vi "rsscope_core_global.vi"() -> ()   [LabVIEW 2018] (continued)
"Data Type"=0, "Command"="SENS:SOUR", "Access"=2, "Range Table"="rsscope_rngIntExt", "Read Callback"="", "Write Callback"="", "Supported Models"="", "Instrument Options"="B4", "Flags"=0, "Help"="Enables the use of the external reference signal instead of the internal OCXO reference.\n\nAvailable Repeated Capabilities:\nNone\n\nRemote-control command(s):\nSENSe[:ROSCillator]:SOURce"}, {"Level"=2, "Class Only"=FALSE, "Identifier"="RSSCOPE_ATTR_REF_OSCILLATOR_FREQUENCY", "Descriptive Name"="Ref Oscillator Frequency", "Data Type"=1, "Command"="SENS:EXT:FREQ", "Access"=2, "Range Table"="rsscope_rngExtOscFreq", "Read Callback"="", "Write Callback"="", "Supported Models"="", "Instrument Options"="B4", "Flags"=0, "Help"="Sets the frequency of an external reference input signal that is connected to the external reference input on the rear panel.\n\nNote: Increment is 1e+6 Hz.\n\nAvailable Repeated Capabilities:\nNone\n\nRemote-control command(s):\nSENSe[:ROSCillator]:EXTernal:FREQuency"}, {"Level"=1, "Class Only"=TRUE, "Identifier"="", "Descriptive Name"="Probe", "Data Type"=0, "Command"="", "Access"=0, "Range Table"="", "Read Callback"="", "Write Callback"="", "Supported Models"="", "Instrument Options"="", "Flags"=0, "Help"="This class contains attributes that configure the probe subsystem."}, {"Level"=2, "Class Only"=FALSE, "Identifier"="RSSCOPE_ATTR_PROBE_STATE", "Descriptive Name"="Probe State", "Data Type"=0, "Command"="PROB{Channel}:SET:STAT?", "Access"=0, "Range Table"="rsscope_rngProbeState", "Read Callback"="", "Write Callback"="", "Supported Models"="", "Instrument Options"="", "Flags"=0, "Help"="Queries if the probe at the specified input channel is active (detected) or not active (not detected). To switch the probe on, use attribute RSSCOPE_ATTR_CHANNEL_ENABLED.\n\nAvailable Repeated Capabilities:\nChannel: CH1, CH2, CH3, CH4, CHExt\r\n\nRemote-control command(s):\nPROBe<m>:SETup:STATe?"}, {"Level"=2, "Class Only"=FALSE, "Identifier"="RSSCOPE_ATTR_PROBE_TYPE", "Descriptive Name"="Probe Type", "Data Type"=2, "Command"="PROB{Channel}:SET:TYPE?", "Access"=0, "Range Table"="", "Read Callback"="", "Write Callback"="", "Supported Models"="", "Instrument Options"="", "Flags"=0, "Help"="Queries the type of the probe.\n\nAvailable Repeated Capabilities:\nChannel: CH1, CH2, CH3, CH4, CHExt\r\n\nRemote-control command(s):\nPROBe<m>:SETup:TYPE?"}, {"Level"=2, "Class Only"=FALSE, "Identifier"="RSSCOPE_ATTR_PROBE_NAME", "Descriptive Name"="Probe Name", "Data Type"=2, "Command"="PROB{Channel}:SET:NAME?", "Access"=0, "Range Table"="", "Read Callback"="", "Write Callback"="", "Supported Models"="", "Instrument Options"="", "Flags"=0, "Help"="Queries the name of the probe.\n\nAvailable Repeated Capabilities:\nChannel: CH1, CH2, CH3, CH4, CHExt\r\n\nRemote-control command(s):\nPROBe<m>:SETup:NAME?"}, {"Level"=2, "Class Only"=FALSE, "Identifier"="RSSCOPE_ATTR_PROBE_INPUT_IMPEDANCE", "Descriptive Name"="Probe Input Impedance", "Data Type"=1, "Command"="PROB{Channel}:SET:IMP?", "Access"=0, "Range Table"="", "Read Callback"="", "Write Callback"="", "Supported Models"="", "Instrument Options"="", "Flags"=0, "Help"="Queries the termination of the probe.\n\nAvailable Repeated Capabilities:\nChannel: CH1, CH2, CH3, CH4, CHExt\r\n\nRemote-control command(s):\nPROBe<m>:SETup:IMPedance?"}, {"Level"=2, "Class Only"=FALSE, "Identifier"="RSSCOPE_ATTR_PROBE_INPUT_CAPACITANCE", "Descriptive Name"="Probe Input Capacitance", "Data Type"=1, "Command"="PROB{Channel}:SET:CAP?", "Access"=0, "Range Table"="", "Read Callback"="", "Write Callback"="", "Supported Models"="", "Instrument Options"="", "Flags"=0, "Help"="Queries the input capacitance of the probe.\n\nAvailable Repeated Capabilities:\nChannel: CH1, CH2, CH3, CH4, CHExt\r\n\nRemote-control command(s):\nPROBe<m>:SETup:CAPacitance?"}, {"Level"=2, "Class Only"=FALSE, "Identifier"="RSSCOPE_ATTR_PROBE_ATTENUATION", "Descriptive Name"="Probe Attenuation", "Data Type"=1, "Command"="PROB{Channel}:SET:ATT?", "Access"=0, "Range Table"="", "Read Callback"="", "Write Callback"="", "Supported Models"="", "Instrument Options"="", "Flags"=0, "Help"="Queries the attenuation of the probe.\n\nAvailable Repeated Capabilities:\nChannel: CH1, CH2, CH3, CH4, CHExt\r\n\nRemote-control command(s):\nPROBe<m>:SETup:ATTenuation[:AUTO]?"}, {"Level"=2, "Class Only"=FALSE, "Identifier"="RSSCOPE_ATTR_PROBE_BANDWIDTH", "Descriptive Name"="Probe Bandwidth", "Data Type"=1, "Command"="PROB{Channel}:SET:BANDwidth?", "Access"=0, "Range Table"="", "Read Callback"="", "Write Callback"="", "Supported Models"="", "Instrument Options"="", "Flags"=0, "Help"="Queries the bandwidth of the probe.\n\nAvailable Repeated Capabilities:\nChannel: CH1, CH2, CH3, CH4, CHExt\r\n\nRemote-control command(s):\nPROBe<m>:SETup:BANDwidth?"}, {"Level"=2, "Class Only"=FALSE, "Identifier"="RSSCOPE_ATTR_PROBE_SET_OFFSET_TO_MEAN", "Descriptive Name"="Probe Set Offset To Mean", "Data Type"=4, "Command"="PROB{Channel}:SET:OFFS:TOM", "Access"=1, "Range Table"="", "Read Callback"="", "Write Callback"="", "Supported Models"="", "Instrument Options"="", "Flags"=1, "Help"="Performs an automatic compensation for a DC component of the specified input signal using the result of a background mean measurement.\n\nAvailable Repeated Capabilities:\nChannel: CH1, CH2, CH3, CH4, CHExt\r\n\nRemote-control command(s):\nPROBe<m>:SETup:OFFSet:TOMean"}, {"Level"=2, "Class Only"=FALSE, "Identifier"="RSSCOPE_ATTR_PROBE_DEGAUSS", "Descriptive Name"="Probe Degauss", "Data Type"=4, "Command"="PROB{Channel}:SET:DEG", "Access"=1, "Range Table"="", "Read Callback"="", "Write Callback"="", "Supported Models"="", "Instrument Options"="", "Flags"=0, "Help"="Demagnetizes the core if it has been magnetized by switching the power on and off, or by an excessive input. Always carry out demagnetizing before measurement. The demagnetizing process takes about one second.\n\nAvailable Repeated Capabilities:\nChannel: CH1, CH2, CH3, CH4, CHExt\r\n\nRemote-control command(s):\nPROBe<m>:SETup:DEGauss"}, {"Level"=2, "Class Only"=FALSE, "Identifier"="RSSCOPE_ATTR_PROBE_AUTO_ZERO", "Descriptive Name"="Probe Auto Zero", "Data Type"=4, "Command"="PROB{Channel}:SET:OFFS:AZER", "Access"=1, "Range Table"="", "Read Callback"="", "Write Callback"="", "Supported Models"="", "Instrument Options"="", "Flags"=1, "Help"="Performs an automatic correction of the zero error. If the DUT is ground-referenced, the Auto Zero function can improve the measurement results.\n\nAvailable Repeated Capabilities:\nChannel: CH1, CH2, CH3, CH4, CHExt\r\n\nRemote-control command(s):\nPROBe<m>:SETup:OFFSet:AZERo"}, {"Level"=2, "Class Only"=FALSE, "Identifier"="RSSCOPE_ATTR_PROBE_USE_AUTO_ZERO", "Descriptive Name"="Probe Use Auto Zero", "Data Type"=3, "Command"="PROB{Channel}:SET:OFFS:USE", "Access"=2, "Range Table"="", "Read Callback"="", "Write Callback"="", "Supported Models"="", "Instrument Options"="", "Flags"=0, "Help"="Includes the AutoZero offset in measurement results.\n\nAvailable Repeated Capabilities:\nChannel: CH1, CH2, CH3, CH4, CHExt\r\n\nRemote-control command(s):\nPROBe<m>:SETup:OFFSet:USEautozero"}, {"Level"=2, "Class Only"=FALSE, "Identifier"="RSSCOPE_ATTR_PROBE_ZERO_ADJUST_VALUE", "Descriptive Name"="Probe Zero Adjust Value", "Data Type"=1, "Command"="PROB{Channel}:SET:OFFS:ZADJ", "Access"=2, "Range Table"="RsScope_rngProbeZeroAdjustValue", "Read Callback"="", "Write Callback"="", "Supported Models"="", "Instrument Options"="", "Flags"=0, "Help"="Set the waveform to zero position. It corrects the effect of a voltage offset or temperature drift.\n\nAvailable Repeated Capabilities:\nChannel: CH1, CH2, CH3, CH4, CHExt\r\n\nRemote-control command(s):\nPROBe<m>:SETup:OFFSet:ZADJust"}, {"Level"=2, "Class Only"=FALSE, "Identifier"="RSSCOPE_ATTR_PROBE_SAVE_TO_PROBE", "Descriptive Name"="Probe Save To Probe", "Data Type"=4, "Command"="PROB{Channel}:SET:OFFS:STPR", "Access"=1, "Range Table"="", "Read Callback"="", "Write Callback"="", "Supported Models"="", "Instrument Options"="", "Flags"=0, "Help"="Saves the zero adjust value in the probe box. If you connect the probe to another channel or to another R&S RTx oscilloscope, the value is read out again.\n\nAvailable Repeated Capabilities:\nChannel: CH1, CH2, CH3, CH4, CHExt\r\n\nRemote-control command(s):\nPROBe<m>:SETup:OFFSet:STPRobe"}, {"Level"=2, "Class Only"=FALSE, "Identifier"="RSSCOPE_ATTR_PROBE_MICRO_BUTTON_ACTION", "Descriptive Name"="Probe Micro Button Action", "Data Type"=0, "Command"="PROB{Channel}:SET:MODE", "Access"=2, "Range Table"="rsscope_rngProbeButtonAction", "Read Callback"="", "Write Callback"="", "Supported Models"="", "Instrument Options"="", "Flags"=0, "Help"="Select the action that is started with the micro button on the probe head.\n\nAvailable Repeated Capabilities:\nChannel: CH1, CH2, CH3, CH4, CHExt\r\n\nRemote-control command(s):\nPROBe<m>:SETup:MODE"}, {"Level"=2, "Class Only"=FALSE, "Identifier"="RSSCOPE_ATTR_PROBE_SOFTWARE_VERSION", "Descriptive Name"="Probe Software Version", "Data Type"=2, "Command"="PROB{Channel}:ID:SWV?", "Access"=0, "Range Table"="", "Read Callback"="", "Write Callback"="", "Supported Models"="", "Instrument Options"="", "Flags"=0, "Help"="Queries the version of the probe firmware.\n\nAvailable Repeated Capabilities:\nChannel: CH1, CH2, CH3, CH4, CHExt\r\n\nRemote-control command(s):\nPROBe<m>:ID:SWVersion?"}, {"Level"=2, "Class Only"=FALSE, "Identifier"="RSSCOPE_ATTR_PROBE_PRODUCTION_DATE", "Descriptive Name"="Probe Production Date", "Data Type"=2, "Command"="PROB{Channel}:ID:PRD?", "Access"=0, "Range Table"="", "Read Callback"="", "Write Callback"="", "Supported Models"="", "Instrument Options"="", "Flags"=0, "Help"="Queries the production date of the probe.\n\nAvailable Repeated Capabilities:\nChannel: CH1, CH2, CH3, CH4, CHExt\r\n\nRemote-control command(s):\nPROBe<m>:ID:PRDate?"}, {"Level"=2, "Class Only"=FALSE, "Identifier"="RSSCOPE_ATTR_PROBE_PART_NUMBER", "Descriptive Name"="Probe Part Number", "Data Type"=2, "Command"="PROB{Channel}:ID:PART?", "Access"=0, "Range Table"="", "Read Callback"="", "Write Callback"="", "Supported Models"="", "Instrument Options"="", "Flags"=0, "Help"="Queries the R&S part number of the probe.\n\nAvailable Repeated Capabilities:\nChannel: CH1, CH2, CH3, CH4, CHExt\r\n\nRemote-control command(s):\nPROBe<m>:ID:PARTnumber?"}, {"Level"=2, "Class Only"=FALSE, "Identifier"="RSSCOPE_ATTR_PROBE_SERIAL_NUMBER", "Descriptive Name"="Probe Serial Number", "Data Type"=2, "Command"="PROB{Channel}:ID:SRN?", "Access"=0, "Range Table"="", "Read Callback"="", "Write Callback"="", "Supported Models"="", "Instrument Options"="", "Flags"=0, "Help"="Queries the serial number of the probe.\n\nAvailable Repeated Capabilities:\nChannel: CH1, CH2, CH3, CH4, CHExt\r\n\nRemote-control command(s):\nPROBe<m>:ID:SRNumber?"}, {"Level"=2, "Class Only"=FALSE, "Identifier"="RSSCOPE_ATTR_PROBE_FIRMWARE_PATH", "Descriptive Name"="Probe Firmware Path", "Data Type"=2, "Command"="PROB{Channel}:SERV:FW:PATH", "Access"=2, "Range Table"="", "Read Callback"="", "Write Callback"="", "Supported Models"="", "Instrument Options"="", "Flags"=0, "Help"="Configures the path and file name of the update package.\n\nAvailable Repeated Capabilities:\nChannel: CH1, CH2, CH3, CH4, CHExt\r\n\nRemote-control command(s):\nPROBe<m>:SERVice:FW:PATH"}, {"Level"=2, "Class Only"=FALSE, "Identifier"="RSSCOPE_ATTR_PROBE_FIRMWARE_UPDATE", "Descriptive Name"="Probe Firmware Update", "Data Type"=4, "Command"="PROB{Channel}:SERV:FW:FLAS", "Access"=1, "Range Table"="", "Read Callback"="", "Write Callback"="", "Supported Models"="", "Instrument Options"="", "Flags"=0, "Help"="Starts the update of the probe firmware.\n\nAvailable Repeated Capabilities:\nChannel: CH1, CH2, CH3, CH4, CHExt\r\n\nRemote-control command(s):\nPROBe<m>:SERVice:FW:FLASh"}, {"Level"=2, "Class Only"=FALSE, "Identifier"="RSSCOPE_ATTR_PROBE_FIRMWARE_UPDATE_STATUS", "Descriptive Name"="Probe Firmware Update Status", "Data Type"=0, "Command"="PROB{Channel}:SERV:STAT?", "Access"=0, "Range Table"="rsscope_rngProbeFirmwareUpdateStatus", "Read Callback"="", "Write Callback"="", "Supported Models"="", "Instrument Options"="", "Flags"=0, "Help"="Queries the update status of the probe firmware.\n\nAvailable Repeated Capabilities:\nChannel: CH1, CH2, CH3, CH4, CHExt\r\n\nRemote-control command(s):\nPROBe<m>:SERVice:STATe?"}, {"Level"=2, "Class Only"=FALSE, "Identifier"="RSSCOPE_ATTR_PROBE_SELFTEST", "Descriptive Name"="Probe Selftest", "Data Type"=4, "Command"="PROB{Channel}:SERV:STES:RUN", "Access"=1, "Range Table"="", "Read Callback"="", "Write Callback"="", "Supported Models"="", "Instrument Options"="", "Flags"=0, "Help"="Starts the selftest of the probe connected to the specified channel input.\n\nAvailable Repeated Capabilities:\nChannel: CH1, CH2, CH3, CH4, CHExt\r\n\nRemote-control command(s):\nPROBe<m>:SERVice:STESt:RUN"}, {"Level"=2, "Class Only"=FALSE, "Identifier"="RSSCOPE_ATTR_PROBE_SELFTEST_STATUS", "Descriptive Name"="Probe Selftest Status", "Data Type"=0, "Command"="PROB{Channel}:SERV:STES:STAT?", "Access"=0, "Range Table"="rsscope_rngProbeSelftestStatus", "Read Callback"="", "Write Callback"="", "Supported Models"="", "Instrument Options"="", "Flags"=0, "Help"="Queries the status of a probe selftest for the specified channel input. When the selftest has finished, the status is passed or failed, otherwise it is undefined.\n\nAvailable Repeated Capabilities:\nChannel: CH1, CH2, CH3, CH4, CHExt\r\n\nRemote-control command(s):\nPROBe<m>:SERVice:STESt:STATus?"}, {"Level"=2, "Class Only"=FALSE, "Identifier"="RSSCOPE_ATTR_PROBE_DETECTION_MODE", "Descriptive Name"="Probe Detection Mode", "Data Type"=0, "Command"="PROB{Channel}:SET:ATT:MODE", "Access"=2, "Range Table"="rsscope_rngAutoManual", "Read Callback"="", "Write Callback"="", "Supported Models"="", "Instrument Options"="", "Flags"=0, "Help"="Sets mode of probe detection.\n\nAvailable Repeated Capabilities:\nChannel: CH1, CH2, CH3, CH4, CHExt\r\n\nRemote-control command(s):\nPROBe<m>:SETup:ATTenuation:MODE"}, {"Level"=2, "Class Only"=FALSE, "Identifier"="RSSCOPE_ATTR_PROBE_ATTENUATION_MANUAL", "Descriptive Name"="Probe Attenuation Manual", "Data Type"=1, "Command"="PROB{Channel}:SET:ATT:MAN", "Access"=2, "Range Table"="rsscope_rngAttenuation", "Read Callback"="", "Write Callback"="", "Supported Models"="", "Instrument Options"="", "Flags"=0, "Help"="Sets the attenuation for the connected probe.\n\nAvailable Repeated Capabilities:\nChannel: CH1, CH2, CH3, CH4, CHExt\r\n\nRemote-control command(s):\nPROBe<m>:SETup:ATTenuation:MANual"}, {"Level"=2, "Class Only"=FALSE, "Identifier"="RSSCOPE_ATTR_PROBE_VERTICAL_UNIT", "Descriptive Name"="Probe Vertical Unit", "Data Type"=0, "Command"="PROB{Channel}:SET:ATT:UNIT", "Access"=2, "Range Table"="rsscope_rngAttUnits", "Read Callback"="", "Write Callback"="", "Supported Models"="", "Instrument Options"="", "Flags"=0, "Help"="Sets the unit for the connected probe type.\n\nAvailable Repeated Capabilities:\nChannel: CH1, CH2, CH3, CH4, CHExt\r\n\nRemote-control command(s):\nPROBe<m>:SETup:ATTenuation:UNIT"}, {"Level"=2, "Class Only"=FALSE, "Identifier"="RSSCOPE_ATTR_PROBE_GAIN_MANUAL", "Descriptive Name"="Probe Gain Manual", "Data Type"=1, "Command"="PROB{Channel}:SET:GAIN:MAN", "Access"=2, "Range Table"="rsscope_rngProbeGainManual", "Read Callback"="", "Write Callback"="", "Supported Models"="", "Instrument Options"="", "Flags"=0, "Help"="Sets the gain of a current probe.\n\nAvailable Repeated Capabilities:\nChannel: CH1, CH2, CH3, CH4, CHExt\r\n\nRemote-control command(s):\nPROBe<m>:SETup:GAIN:MANual"}, {"Level"=2, "Class Only"=FALSE, "Identifier"="RSSCOPE_ATTR_DETECTED_PROBE_GAIN", "Descriptive Name"="Detected Probe Gain", "Data Type"=1, "Command"="PROB{Channel}:SET:GAIN:AUTO?", "Access"=0, "Range Table"="", "Read Callback"="", "Write Callback"="", "Supported Models"="", "Instrument Options"="", "Flags"=0, "Help"="Returns the gain of an automatically detected current probe.\n\nAvailable Repeated Capabilities:\nChannel: CH1, CH2, CH3, CH4, CHExt\r\n\nRemote-control command(s):\nPROBe<m>:SETup:GAIN:AUTO?"}, {"Level"=2, "Class Only"=FALSE, "Identifier"="RSSCOPE_ATTR_PROBE_PREDEFINED_CURRENT_PROBE", "Descriptive Name"="Probe Predefined Current Probe", "Data Type"=0, "Command"="PROB{Channel}:SET:ATT:DEFP", "Access"=2, "Range Table"="rsscope_rngProbePredefinedCurrent", "Read Callback"="", "Write Callback"="", "Supported Models"="", "Instrument Options"="", "Flags"=0, "Help"="This attribute select the predefined current probe. Current probes are not recognized automatically but the parameters of R&S current probes (R&S RT-ZCxx) are known to the instrument.\n\nAvailable Repeated Capabilities:\nChannel: CH1, CH2, CH3, CH4, CHExt\r\n\nRemote-control command(s):\nPROBe<m>:SETup:ATTenuation:DEFProbe"}, {"Level"=2, "Class Only"=FALSE, "Identifier"="RSSCOPE_ATTR_PROBE_PREDEFINED_TEKTRONICS_PROBE", "Descriptive Name"="Probe Predefined Tektronics Probe", "Data Type"=0, "Command"="PROB{Channel}:SET:ATT:TDEF", "Access"=2, "Range Table"="RsScope_rngProbePredefinedTektronics", "Read Callback"="", "Write Callback"="", "Supported Models"="", "Instrument Options"="", "Flags"=0, "Help"="Selects the Tektronics probe that is connected to the R&S RT-Z2T adapter.\n\nAvailable Repeated Capabilities:\nChannel: CH1, CH2, CH3, CH4, CHExt\r\n\nRemote-control command(s):\nPROBe<m>:SETup:ATTenuation:TDEFprobe"}, {"Level"=2, "Class Only"=FALSE, "Identifier"="RSSCOPE_ATTR_PROBE_MODE", "Descriptive Name"="Probe Mode", "Data Type"=0, "Command"="PROB{Channel}:SET:PRM", "Access"=2, "Range Table"="RsScope_rngModularProbeMode", "Read Callback"="", "Write Callback"="", "Supported Models"="", "Instrument Options"="", "Flags"=0, "Help"="Sets the measurement mode of the modular probe.\n\nAvailable Repeated Capabilities:\nChannel: CH1, CH2, CH3, CH4, CHExt\r\n\nRemote-control command(s):\nPROBe<m>:SETup:PRMode"}, {"Level"=2, "Class Only"=FALSE, "Identifier"="RSSCOPE_ATTR_PROBE_DM_OFFSET", "Descriptive Name"="Probe DM Offset", "Data Type"=1, "Command"="PROB{Channel}:SET:DMOF", "Access"=2, "Range Table"="RsScope_rngProbeOffset", "Read Callback"="", "Write Callback"="", "Supported Models"="", "Instrument Options"="", "Flags"=0, "Help"="Sets the differential offset to compensate a DC voltage applied to the positive and the negative input terminal.\n\nAvailable Repeated Capabilities:\nChannel: CH1, CH2, CH3, CH4, CHExt\r\n\nRemote-control command(s):\nPROBe<m>:SETup:DMOFfset"}, {"Level"=2, "Class Only"=FALSE, "Identifier"="RSSCOPE_ATTR_PROBE_CM_OFFSET", "Descriptive Name"="Probe CM Offset", "Data Type"=1, "Command"="PROB{Channel}:SET:CMOF", "Access"=2, "Range Table"="", "Read Callback"="", "Write Callback"="", "Supported Models"="", "Instrument Options"="", "Flags"=0, "Help"="Sets the common-mode offset. The setting is only available for differential probes.\n\nAvailable Repeated Capabilities:\nChannel: CH1, CH2, CH3, CH4, CHExt\r\n\nRemote-control command(s):\nPROBe<m>:SETup:CMOFfset"}, {"Level"=2, "Class Only"=FALSE, "Identifier"="RSSCOPE_ATTR_PROBE_POSITIVE_OFFSET", "Descriptive Name"="Probe Positive Offset", "Data Type"=1, "Command"="PROB{Channel}:SET:POFF", "Access"=2, "Range Table"="RsScope_rngProbeOffset", "Read Callback"="", "Write Callback"="", "Supported Models"="", "Instrument Options"="", "Flags"=0, "Help"="Sets the positive offset to compensate a DC voltage applied to the positive input terminal (Vp) referenced to ground.\n\nAvailable Repeated Capabilities:\nChannel: CH1, CH2, CH3, CH4, CHExt\r\n\nRemote-control command(s):\nPROBe<m>:SETup:POFFset"}, {"Level"=2, "Class Only"=FALSE, "Identifier"="RSSCOPE_ATTR_PROBE_NEGATIVE_OFFSET", "Descriptive Name"="Probe Negative Offset", "Data Type"=1, "Command"="PROB{Channel}:SET:NOFF", "Access"=2, "Range Table"="RsScope_rngProbeOffset", "Read Callback"="", "Write Callback"="", "Supported Models"="", "Instrument Options"="", "Flags"=0, "Help"="Sets the negative offset to compensate a DC voltage applied to the negative input terminal (Vp) referenced to ground.\n\nAvailable Repeated Capabilities:\nChannel: CH1, CH2, CH3, CH4, CHExt\r\n\nRemote-control command(s):\nPROBe<m>:SETup:NOFFset"}, {"Level"=2, "Class Only"=FALSE, "Identifier"="RSSCOPE_ATTR_PROBE_ATTENUATOR_ZA15", "Descriptive Name"="Probe Attenuator ZA15", "Data Type"=3, "Command"="PROB{Channel}:SET:ZAXV", "Access"=2, "Range Table"="", "Read Callback"="", "Write Callback"="", "Supported Models"="", "Instrument Options"="", "Flags"=0, "Help"="If you use the external attenuator R&S RT-ZA15 together with one of the differential active probes R&S RT-ZD10/20/30, enable RT-ZA15 to include the external attenuation in the measurements.\n\nAvailable Repeated Capabilities:\nChannel: CH1, CH2, CH3, CH4, CHExt\r\n\nRemote-control command(s):\nPROBe<m>:SETup:ZAXV"}, {"Level"=2, "Class Only"=FALSE, "Identifier"="RSSCOPE_ATTR_PROBE_TERMINATION_VOLTAGE_MODE", "Descriptive Name"="Probe Termination Voltage Mode", "Data Type"=0, "Command"="PROB{Channel}:SET:TERM:MODE", "Access"=2, "Range Table"="rsscope_rngAutoManual", "Read Callback"="", "Write Callback"="", "Supported Models"="", "Instrument Options"="", "Flags"=0, "Help"="Setting the termination voltage is relevant if you use the R&S RT-ZMA40 SMA module.\nYou can set a termination voltage to correct the internal 50  termination of the SMA module by the common mode voltage. To control the termination voltage by the instrument, connect the VT terminal of the R&S RT-ZM probe amplifier to the VT terminal of the SMA module using the red DC lead (see R&S RT-ZM User Manual).\n\nAvailable Repeated Capabilities:\nChannel: CH1, CH2, CH3, CH4, CHExt\r\n\nRemote-control command(s):\nPROBe<m>:SETup:TERM:MODE"}, {"Level"=2, "Class Only"=FALSE, "Identifier"="RSSCOPE_ATTR_PROBE_TERMINATION_VOLTAGE_STATE", "Descriptive Name"="Probe Termination Voltage State", "Data Type"=3, "Command"="PROB{Channel}:SET:TERM:STAT", "Access"=2, "Range Table"="", "Read Callback"="", "Write Callback"="", "Supported Models"="", "Instrument Options"="", "Flags"=0, "Help"="Activates the instrument control of the termination voltage.\n\nAvailable Repeated Capabilities:\nChannel: CH1, CH2, CH3, CH4, CHExt\r\n\nRemote-control command(s):\nPROBe<m>:SETup:TERM:STATe"}, {"Level"=2, "Class Only"=FALSE, "Identifier"="RSSCOPE_ATTR_PROBE_TERMINATION_VOLTAGE_ADJUSTMENT", "Descriptive Name"="Probe Termination Voltage Adjustment", "Data Type"=1, "Command"="PROB{Channel}:SET:TERM:ADJ", "Access"=2, "Range Table"="RsScope_rngProbeTerminationVoltageAdjustment", "Read Callback"="", "Write Callback"="", "Supported Models"="", "Instrument Options"="", "Flags"=0, "Help"="Sets the voltage to be used for termination correction.\n\nAvailable Repeated Capabilities:\nChannel: CH1, CH2, CH3, CH4, CHExt\r\n\nRemote-control command(s):\nPROBe<m>:SETup:TERM:ADJust"}, {"Level"=2, "Class Only"=FALSE, "Identifier"="RSSCOPE_ATTR_PROBE_TERMINATION_VOLTAGE_MEASURE", "Descriptive Name"="Probe Termination Voltage Measure", "Data Type"=1, "Command"="PROB{Channel}:SET:TERM:MEAS?", "Access"=0, "Range Table"="", "Read Callback"="", "Write Callback"="", "Supported Models"="", "Instrument Options"="", "Flags"=0, "Help"="Returns the measured common mode voltage.\n\nAvailable Repeated Capabilities:\nChannel: CH1, CH2, CH3, CH4, CHExt\r\n\nRemote-control command(s):\nPROBe<m>:SETup:TERM:MEASure?"}, {"Level"=2, "Class Only"=FALSE, "Identifier"="RSSCOPE_ATTR_PROBE_COUPLING_AC", "Descriptive Name"="Probe Coupling AC", "Data Type"=3, "Command"="PROB{Channel}:SET:ACC", "Access"=2, "Range Table"="", "Read Callback"="", "Write Callback"="", "Supported Models"="", "Instrument Options"="", "Flags"=0, "Help"="Enables AC coupling in the R&S RT-ZPR20 probe, which removes DC and very lowfrequency components. The R&S RT-ZPR20 probe requires 50  input termination, for which the channel AC coupling is not available. The probe setting allows AC coupling also at 50  inputs.\n\nAvailable Repeated Capabilities:\nChannel: CH1, CH2, CH3, CH4, CHExt\r\n\nRemote-control command(s):\nPROBe<m>:SETup:ACCoupling"}, {"Level"=2, "Class Only"=FALSE, "Identifier"="RSSCOPE_ATTR_PROBE_DEEMBEDDING_MODE", "Descriptive Name"="Probe Deembedding Mode", "Data Type"=0, "Command"="PROB{Channel}:DEEM:PMOD", "Access"=2, "Range Table"="RsScope_rngModularProbeMode", "Read Callback"="", "Write Callback"="", "Supported Models"="", "Instrument Options"="", "Flags"=0, "Help"="Selects a probe mode for deembedding.\n\nAvailable Repeated Capabilities:\nChannel: CH1, CH2, CH3, CH4, CHExt\r\n\nRemote-control command(s):\nPROBe<m>:DEEMbedding:PMODe"}, {"Level"=2, "Class Only"=FALSE, "Identifier"="RSSCOPE_ATTR_PROBE_DEEMBEDDING_SELECT_TIP_MODULE", "Descriptive Name"="Probe Deembedding Select Tip Module", "Data Type"=0, "Command"="PROB{Channel}:DEEM:TIPM", "Access"=2, "Range Table"="RsScope_rngProbeTipModule", "Read Callback"="", "Write Callback"="", "Supported Models"="", "Instrument Options"="", "Flags"=0, "Help"="Selects the tip module that is used for measurement.\n\nAvailable Repeated Capabilities:\nChannel: CH1, CH2, CH3, CH4, CHExt\r\n\nRemote-control command(s):\nPROBe<m>:DEEMbedding:TIPModule[:SELect]"}, {"Level"=2, "Class Only"=FALSE, "Identifier"="RSSCOPE_ATTR_PROBE_DEEMBEDDING_CUSTOM_TIP_FILE", "Descriptive Name"="Probe Deembedding Custom Tip File", "Data Type"=2, "Command"="PROB{Channel}:DEEM:TIPM:CSPF", "Access"=2, "Range Table"="", "Read Callback"="", "Write Callback"="", "Supported Models"="", "Instrument Options"="", "Flags"=0, "Help"="Sets the file name, file format and path of the S-parameter file, and loads the S-parameters of user-defined tip modules. Parameter is string with path, file name, and extension.\n\nAvailable Repeated Capabilities:\nChannel: CH1, CH2, CH3, CH4, CHExt\r\n\nRemote-control command(s):\nPROBe<m>:DEEMbedding:TIPModule:CSPFile"}, {"Level"=2, "Class Only"=FALSE, "Identifier"="RSSCOPE_ATTR_PROBE_DEEMBEDDING_ZMA30_SELECT_TIP_SUBMODULE", "Descriptive Name"="Probe Deembedding ZMA30 Select Tip Submodule", "Data Type"=0, "Command"="PROB{Channel}:DEEM:TIPM:ZMA30:SUBM", "Access"=2, "Range Table"="RsScope_rngProbeDeembeddingZMA30SelectTipDistance", "Read Callback"="", "Write Callback"="", "Supported Models"="", "Instrument Options"="", "Flags"=0, "Help"="Selects the space between the pins of the RT-ZMA30 module tip.\n\nAvailable Repeated Capabilities:\nChannel: CH1, CH2, CH3, CH4, CHExt\r\n\nRemote-control command(s):\nPROBe<m>:DEEMbedding:TIPModule:ZMA<n>:SUBModule"}, {"Level"=2, "Class Only"=FALSE, "Identifier"="RSSCOPE_ATTR_PROBE_DEEMBEDDING_ZMA40_SELECT_TIP_SUBMODULE", "Descriptive Name"="Probe Deembedding ZMA40 Select Tip Submodule", "Data Type"=0, "Command"="PROB{Channel}:DEEM:TIPM:ZMA40:SUBM", "Access"=2, "Range Table"="RsScope_rngProbeDeembeddingZMA40SelectTipSubmodule", "Read Callback"="", "Write Callback"="", "Supported Models"="", "Instrument Options"="", "Flags"=0, "Help"="Choose the used submodule: semi-rigid cables or none.\n\nAvailable Repeated Capabilities:\nChannel: CH1, CH2, CH3, CH4, CHExt\r\n\nRemote-control command(s):\nPROBe<m>:DEEMbedding:TIPModule:ZMA<n>:SUBModule"}, {"Level"=2, "Class Only"=FALSE, "Identifier"="RSSCOPE_ATTR_PROBE_DEEMBEDDING_BANDWIDTH", "Descriptive Name"="Probe Deembedding Bandwidth", "Data Type"=1, "Command"="PROB{Channel}:DEEM:BAND", "Access"=2, "Range Table"="RsScope_rngProbeDeembeddingBandwidth", "Read Callback"="", "Write Callback"="", "Supported Models"="", "Instrument Options"="", "Flags"=0, "Help"="Sets the maximum bandwidth until which the signal is corrected. This maximum value is the minimum bandwidth value of probe, probe tip and oscilloscope bandwidth, and can not be higher than the highest frequency in a used S-parameter file. Consider that most tip modules support the full bandwidth of the probe amplifier, but some tip modules have limited bandwidth.\n\nAvailable Repeated Capabilities:\nChannel: CH1, CH2, CH3, CH4, CHExt\r\n\nRemote-control command(s):\nPROBe<m>:DEEMbedding:BANDwidth"}, {"Level"=2, "Class Only"=FALSE, "Identifier"="RSSCOPE_ATTR_PROBE_DEEMBEDDING_PROBING_MODE", "Descriptive Name"="Probe Deembedding Probing Mode", "Data Type"=0, "Command"="PROB{Channel}:DEEM:MODE", "Access"=2, "Range Table"="RsScope_rngDeembeddingProbingMode", "Read Callback"="", "Write Callback"="", "Supported Models"="", "Instrument Options"="", "Flags"=0, "Help"="Sets the probing mode.\n\nAvailable Repeated Capabilities:\nChannel: CH1, CH2, CH3, CH4, CHExt\r\n\nRemote-control command(s):\nPROBe<m>:DEEMbedding:MODE"}, {"Level"=2, "Class Only"=FALSE, "Identifier"="RSSCOPE_ATTR_PROBE_DEEMBEDDING_REMOVE_PROBE_LOADING", "Descriptive Name"="Probe Deembedding Remove Probe Loading", "Data Type"=3, "Command"="PROB{Channel}:DEEM:REMP", "Access"=2, "Range Table"="", "Read Callback"="", "Write Callback"="", "Supported Models"="", "Instrument Options"="", "Flags"=0, "Help"="Removes the loading of the probe if RSSCOPE_ATTR_DEEMBEDDING_COMPONENT_MODE is set to PROBing. If the probe loading is removed, you see the signal that would be at the measurement point if the probe&apos;s input impedance is ideal (infinite impedance). Without removing the loading, you see the real signal at the measurement point, including the probe loading.\n\nAvailable Repeated Capabilities:\nChannel: CH1, CH2, CH3, CH4, CHExt\r\n\nRemote-control command(s):\nPROBe<m>:DEEMbedding:REMProbeload"}, {"Level"=2, "Class Only"=FALSE, "Identifier"="RSSCOPE_ATTR_PROBE_DEEMBEDDING_IMPEDANCE_TYPE", "Descriptive Name"="Probe Deembedding Impedance Type", "Data Type"=0, "Command"="PROB{Channel}:DEEM:LOAD", "Access"=2, "Range Table"="RsScope_rngProbeDeembeddingImpedanceType", "Read Callback"="", "Write Callback"="", "Supported Models"="", "Instrument Options"="", "Flags"=0, "Help"="Sets the impedance type of the DUT.\n\nAvailable Repeated Capabilities:\nChannel: CH1, CH2, CH3, CH4, CHExt\r\n\nRemote-control command(s):\nPROBe<m>:DEEMbedding:LOAD[:TYPE]"}, {"Level"=2, "Class Only"=FALSE, "Identifier"="RSSCOPE_ATTR_PROBE_DEEMBEDDING_IMPEDANCE", "Descriptive Name"="Probe Deembedding Impedance", "Data Type"=1, "Command"="PROB{Channel}:DEEM:LOAD:IMP", "Access"=2, "Range Table"="RsScope_rngProbeDeemebeddingImpedance", "Read Callback"="", "Write Callback"="", "Supported Models"="", "Instrument Options"="", "Flags"=0, "Help"="Impedance of the DUT. Shows the default source impedance or sets the user-defined constant impedance value. If an R&S RT-ZM probe is connected, the value depends on the selected probe mode: common mode, differential, or single-ended measurement.\n\nAvailable Repeated Capabilities:\nChannel: CH1, CH2, CH3, CH4, CHExt\r\n\nRemote-control command(s):\nPROBe<m>:DEEMbedding:LOAD:IMPedance"}, {"Level"=2, "Class Only"=FALSE, "Identifier"="RSSCOPE_ATTR_PROBE_DEEMBEDDING_LOAD_S_PARAMETER_FILE", "Descriptive Name"="Probe Deembedding Load S-Parameter File", "Data Type"=2, "Command"="PROB{Channel}:DEEM:LOAD:FILE", "Access"=2, "Range Table"="", "Read Callback"="", "Write Callback"="", "Supported Models"="", "Instrument Options"="", "Flags"=0, "Help"="Sets the file name, file format and path of the S-parameter file, and loads the S-parameters.\nThe attribute is relevant if:\nRSSCOPE_ATTR_PROBE_DEEMBEDDING_PROBING_MODE is Probing\nRSSCOPE_ATTR_PROBE_DEEMBEDDING_REMOVE_PROBE_LOADING is ON\nRSSCOPE_ATTR_PROBE_DEEMBEDDING_IMPEDANCE_TYPE is S1P or S2P\n\nAvailable Repeated Capabilities:\nChannel: CH1, CH2, CH3, CH4, CHExt\r\n\nRemote-control command(s):\nPROBe<m>:DEEMbedding:LOAD:FILE"}, {"Level"=2, "Class Only"=FALSE, "Identifier"="RSSCOPE_ATTR_PROBE_PROBEMETER_COPY_TO_OFFSET", "Descriptive Name"="Probe ProbeMeter Copy To Offset", "Data Type"=4, "Command"="PROB{Channel}:SET:ADV:PMT", "Access"=1, "Range Table"="", "Read Callback"="", "Write Callback"="", "Supported Models"="", "Instrument Options"="", "Flags"=0, "Help"="Sets the measured ProbeMeter value as offset. Make sure that the ProbeMeter is active before you use this attribute. Only available for power rail probes R&S RT-ZPR.\n\nAvailable Repeated Capabilities:\nChannel: CH1, CH2, CH3, CH4, CHExt\r\n\nRemote-control command(s):\nPROBe<m>:SETup:ADVanced:PMToffset"}, {"Level"=2, "Class Only"=FALSE, "Identifier"="RSSCOPE_ATTR_PROBE_RT_ZHD_VOLTAGE_RANGE", "Descriptive Name"="Probe RT-ZHD Voltage Range", "Data Type"=0, "Command"="PROB{Channel}:SET:ADV:RANG", "Access"=2, "Range Table"="RsScope_rngProbeVoltageRange", "Read Callback"="", "Write Callback"="", "Supported Models"="", "Instrument Options"="", "Flags"=0, "Help"="Sets the voltage range of a R&S RT-ZHD probe.\n\nAvailable Repeated Capabilities:\nChannel: CH1, CH2, CH3, CH4, CHExt\r\n\nRemote-control command(s):\nPROBe<m>:SETup:ADVanced:RANGe"}, {"Level"=2, "Class Only"=FALSE, "Identifier"="RSSCOPE_ATTR_PROBE_RT_ZHD_BANDWIDTH_LIMIT", "Descriptive Name"="Probe RT-ZHD Bandwidth Limit", "Data Type"=3, "Command"="PROB{Channel}:SET:ADV:FILT", "Access"=2, "Range Table"="", "Read Callback"="", "Write Callback"="", "Supported Models"="", "Instrument Options"="", "Flags"=0, "Help"="Enables the lowpass filter in the probe control box.\n\nAvailable Repeated Capabilities:\nChannel: CH1, CH2, CH3, CH4, CHExt\r\n\nRemote-control command(s):\nPROBe<m>:SETup:ADVanced:FILTer"}, {"Level"=2, "Class Only"=FALSE, "Identifier"="RSSCOPE_ATTR_PROBE_RT_ZHD_OVERRANGE_BUZZER", "Descriptive Name"="Probe RT-ZHD Overrange Buzzer", "Data Type"=3, "Command"="PROB{Channel}:SET:ADV:AUD", "Access"=2, "Range Table"="", "Read Callback"="", "Write Callback"="", "Supported Models"="", "Instrument Options"="", "Flags"=0, "Help"="Activates the acustic overrange warning in the probe control box.\n\nAvailable Repeated Capabilities:\nChannel: CH1, CH2, CH3, CH4, CHExt\r\n\nRemote-control command(s):\nPROBe<m>:SETup:ADVanced:AUDioverload"}, {"Level"=2, "Class Only"=FALSE, "Identifier"="RSSCOPE_ATTR_PROBE_ADAPTER_TYPE", "Descriptive Name"="Probe Adapter Type", "Data Type"=0, "Command"="PROB{Channel}:SET:ADAP?", "Access"=0, "Range Table"="RsScope_rngProbeAdapterType", "Read Callback"="", "Write Callback"="", "Supported Models"="", "Instrument Options"="", "Flags"=0, "Help"="Queries the adapter status, whether the instrument identified the adapter.\n\nAvailable Repeated Capabilities:\nChannel: CH1, CH2, CH3, CH4, CHExt\r\n\nRemote-control command(s):\nPROBe<m>:SETup:ADAPter?"}, {"Level"=2, "Class Only"=FALSE, "Identifier"="RSSCOPE_ATTR_PROBE_CONVERTER_TYPE", "Descriptive Name"="Probe Converter Type", "Data Type"=0, "Command"="PROB{Channel}:CONV:TYPE?", "Access"=0, "Range Table"="RsScope_rngProbeConverterType", "Read Callback"="", "Write Callback"="", "Supported Models"="RTP", "Instrument Options"="", "Flags"=0, "Help"="Queries the adapter status, whether the instrument identified the adapter.\n\nAvailable Repeated Capabilities:\nChannel: CH1, CH2, CH3, CH4, CHExt\r\n\nRemote-control command(s):\nPROBe<m>:CONVerter:TYPE?"}, {"Level"=2, "Class Only"=FALSE, "Identifier"="RSSCOPE_ATTR_PROBE_RTZ1M_BANDWIDTH_LIMIT", "Descriptive Name"="Probe RT-Z1M Bandwidth Limit", "Data Type"=0, "Command"="PROB{Channel}:CONV:BAND", "Access"=2, "Range Table"="RsScope_rngProbeRTZ1MBandwidthLimit", "Read Callback"="", "Write Callback"="", "Supported Models"="RTP", "Instrument Options"="", "Flags"=0, "Help"="Sets the bandwidth limit of the R&S RT-Z1M probe adapter.\n\nAvailable Repeated Capabilities:\nChannel: CH1, CH2, CH3, CH4, CHExt\r\n\nRemote-control command(s):\nPROBe<m>:CONVerter:BANDwidth"}, {"Level"=2, "Class Only"=FALSE, "Identifier"="RSSCOPE_ATTR_PROBE_RTZ1M_SELF_ALIGN", "Descriptive Name"="Probe RT-Z1M Self Align", "Data Type"=4, "Command"="PROB{Channel}:CONV:SELF", "Access"=1, "Range Table"="", "Read Callback"="", "Write Callback"="", "Supported Models"="RTP", "Instrument Options"="", "Flags"=0, "Help"="Starts the self-alignment of the R&S RT-Z1M probe adapter. When the adapter is detached from the oscilloscope, the values of the self-alignment are discarded, and the original factory-alignment is reloaded. Thus, repeat the self-alignment when you reattach the probe.\n\nAvailable Repeated Capabilities:\nChannel: CH1, CH2, CH3, CH4, CHExt\r\n\nRemote-control command(s):\nPROBe<m>:CONVerter:SELFalign"}, {"Level"=2, "Class Only"=TRUE, "Identifier"="", "Descriptive Name"="Meter", "Data Type"=0, "Command"="", "Access"=0, "Range Table"="", "Read Callback"="", "Write Callback"="", "Supported Models"="", "Instrument Options"="", "Flags"=0, "Help"="This class contains attributes that configure the probe meter subsystem."}, {"Level"=3, "Class Only"=FALSE, "Identifier"="RSSCOPE_ATTR_PMETER_ENABLED", "Descriptive Name"="Probe Meter Enabled", "Data Type"=3, "Command"="PROB{Channel}:PMET:STAT", "Access"=2, "Range Table"="", "Read Callback"="", "Write Callback"="", "Supported Models"="", "Instrument Options"="", "Flags"=0, "Help"="Switches the probe meter on or off.\n\nAvailable Repeated Capabilities:\nChannel: CH1, CH2, CH3, CH4, CHExt\r\n\nRemote-control command(s):\nPROBe<m>:PMETer:STATe"}, {"Level"=3, "Class Only"=FALSE, "Identifier"="RSSCOPE_ATTR_PMETER_VISIBILITY", "Descriptive Name"="Visibility", "Data Type"=3, "Command"="PROB{Channel}:PMET:VIS", "Access"=2, "Range Table"="", "Read Callback"="", "Write Callback"="", "Supported Models"="", "Instrument Options"="", "Flags"=0, "Help"="Activates the integrated R&S ProbeMeter of active R&S probes.\n\nAvailable Repeated Capabilities:\nChannel: CH1, CH2, CH3, CH4, CHExt\r\n\nRemote-control command(s):\nPROBe<m>:PMETer:VISibility"}, {"Level"=3, "Class Only"=FALSE, "Identifier"="RSSCOPE_ATTR_PMETER_DISPLAY_DIFF", "Descriptive Name"="Display Diff", "Data Type"=0, "Command"="PROB:SET:DISP", "Access"=2, "Range Table"="rsscope_rngProbeDisplayDiff", "Read Callback"="", "Write Callback"="", "Supported Models"="", "Instrument Options"="", "Flags"=0, "Help"="Selects the input voltages to be measured by the ProbeMeter of an R&S differential active probe.\n\nAvailable Repeated Capabilities:\nNone\n\nRemote-control command(s):\nPROBe<m>:SETup:DISPlaydiff"}, {"Level"=3, "Class Only"=TRUE, "Identifier"="", "Descriptive Name"="Results", "Data Type"=0, "Command"="", "Access"=0, "Range Table"="", "Read Callback"="", "Write Callback"="", "Supported Models"="", "Instrument Options"="", "Flags"=0, "Help"="Queries selected result."}, {"Level"=4, "Class Only"=FALSE, "Identifier"="RSSCOPE_ATTR_PMETER_MEASUREMENT_COMMON_RESULT", "Descriptive Name"="Common Measurement Result", "Data Type"=1, "Command"="PROB{Channel}:PMET:RES:COMM?", "Access"=0, "Range Table"="", "Read Callback"="", "Write Callback"="", "Supported Models"="", "Instrument Options"="", "Flags"=0, "Help"="Returns the common mode voltage - the mean voltage between the signal sockets and the ground socket.\n\nAvailable Repeated Capabilities:\nChannel: CH1, CH2, CH3, CH4, CHExt\r\n\nRemote-control command(s):\nPROBe<m>:PMETer:RESults:COMMon?"}, {"Level"=4, "Class Only"=FALSE, "Identifier"="RSSCOPE_ATTR_PMATER_MEASUREMENT_DIFFERENTIAL_RESULT", "Descriptive Name"="Differential Measurement Result", "Data Type"=1, "Command"="PROB{Channel}:PMET:RES:DIFF?", "Access"=0, "Range Table"="", "Read Callback"="", "Write Callback"="", "Supported Models"="", "Instrument Options"="", "Flags"=0, "Help"="Returns the differential voltage - the voltage between the positive and negative signal sockets.\n\nAvailable Repeated Capabilities:\nChannel: CH1, CH2, CH3, CH4, CHExt\r\n\nRemote-control command(s):\nPROBe<m>:PMETer:RESults:DIFFerential?"}, {"Level"=4, "Class Only"=FALSE, "Identifier"="RSSCOPE_ATTR_PMETER_MEASUREMENT_POSITIVE_RESULT", "Descriptive Name"="Single Ended Positive Measurement Result", "Data Type"=1, "Command"="PROB{Channel}:PMET:RES:POS?", "Access"=0, "Range Table"="", "Read Callback"="", "Write Callback"="", "Supported Models"="", "Instrument Options"="", "Flags"=0, "Help"="Returns the voltage that is measured between the positive signal socket and the ground.\n\nAvailable Repeated Capabilities:\nChannel: CH1, CH2, CH3, CH4, CHExt\r\n\nRemote-control command(s):\nPROBe<m>:PMETer:RESults:POSitive?"}, {"Level"=4, "Class Only"=FALSE, 
